vi "FeedBack.vi"() -> ()   [LabVIEW 2015]
doc: "This example performs a serial port write and a serial port read. The parameters set for the serial port must match the parameters of the connected instrument or device. The VISA Configure Serial Port VI sets the configuration parameters. The front panel displays the controls used to configure the basic parameters, such as baud rate, data bits, and parity. The VI passes the VISA resource name to other VIs that perform operations on that VISA resource. The VISA Write function sends a command to the serial device and the VISA Read function returns data based on the command. The VISA Close function then closes the reference to the serial device. It is important to close the reference; otherwise, further communication through that port might not be possible."
uses:
  support/Serial - Settings.ctl
  <vilib>/Instr/_visa.llb/VISA Configure Serial Port (Instr).vi
panel:
  out "AzimuthCurrentAngle":u16(knob) caption="ElevationCurrentAngle" scale=0.0..360.0
  in  "Parameter 2":u16
  in  "Azmuth WRITE PORT":refnum<visa-resource-name>="COM1"
  out "AzimuthDirection":string
  out "bytes written 2":u32
  out "Azmuth Encoder":string
  out "bytes read 2":u32
  out "hex integer string 4":string
  out "hex integer string 3":string
  in  "AzimuthRequiredAngle":u16=50
  in  "Azmuth READ PORT":refnum<visa-resource-name>="COM1"
  in  "Elevation WRITE PORT":refnum<visa-resource-name>="COM1"
  out "ElevationDirection":string
  out "bytes written":u32
  out "ElevationCurrentAngle":u16(knob) scale=0.0..360.0
  in  "ElevationRequiredAngle":u16=50
  out "hex integer string 2":string
  out "hex integer string":string
  in  "Parameter":u16
  in  "Combo Box":string(combo)="Get_Position"
  in  "Serial Settings":T1={"baud rate"=9600, "data bits"=8, "parity"=enum."None", "stop bits"=10, "flow control"=0} {"flow control" items=["None"=0, "XON/XOFF"=1, "RTS/CTS"=2, "DTR/DSR"=4]; "stop bits" items=["1.0"=10, "1.5"=15, "2.0"=20]; "data bits" min=5 max=8 step=1; "baud rate" items=["75"=75, "110"=110, "134"=134, "150"=150, "300"=300, "600"=600, "1200"=1200, "1800"=1800, "2400"=2400, "4800"=4800, "7200"=7200, "9600"=9600, "14400"=14400, "19200"=19200, "28800"=28800, "38400"=38400, "56000"=56000, "57600"=57600, "115200"=115200, "128000"=128000, "230400"=230400]}
  out "bytes read":u32
  in  "delay before read (ms)":u32=500
  out "Elevation Encoder":string
  in  "Elevation READ PORT":refnum<visa-resource-name>="COM1"
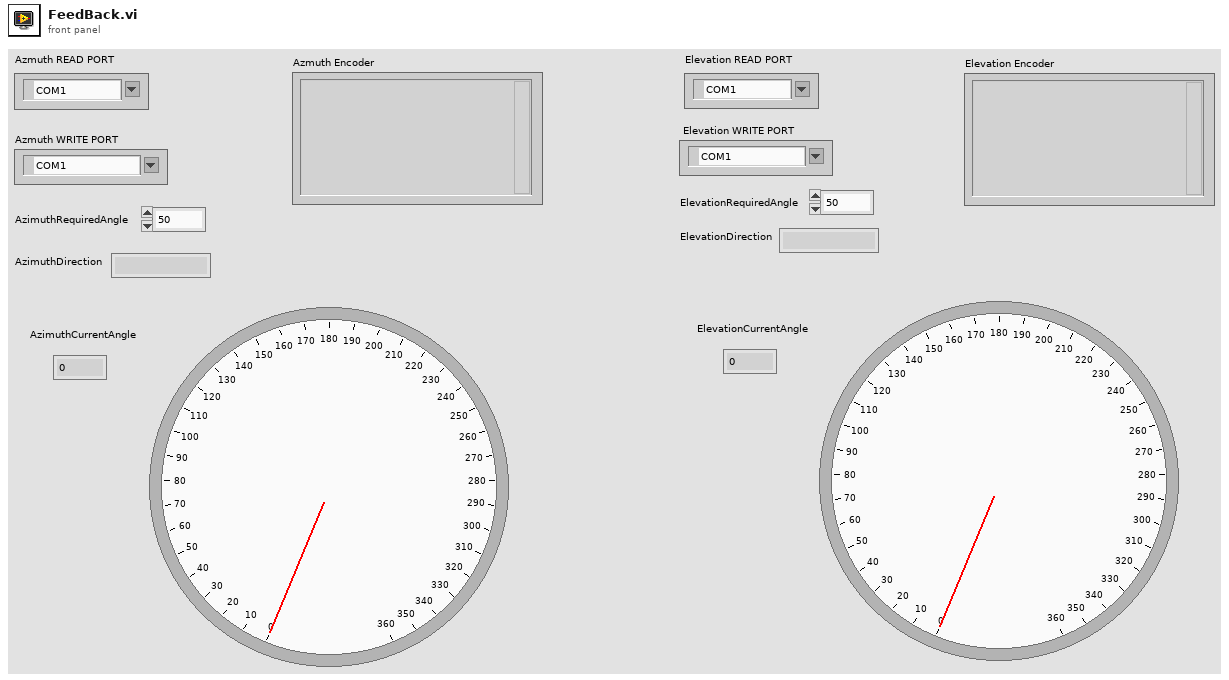
[diagram p1: front panel]
types:
  T1 = typedef "Serial - Settings.ctl" = cluster{"baud rate":u32, "data bits":u16, "parity":enum16{"None", "Odd", "Even", "Mark", "Space"}, "stop bits":u16, "flow control":u16}
  T2 = enum16{"big-endian, network order", "native, host order", "little-endian"}
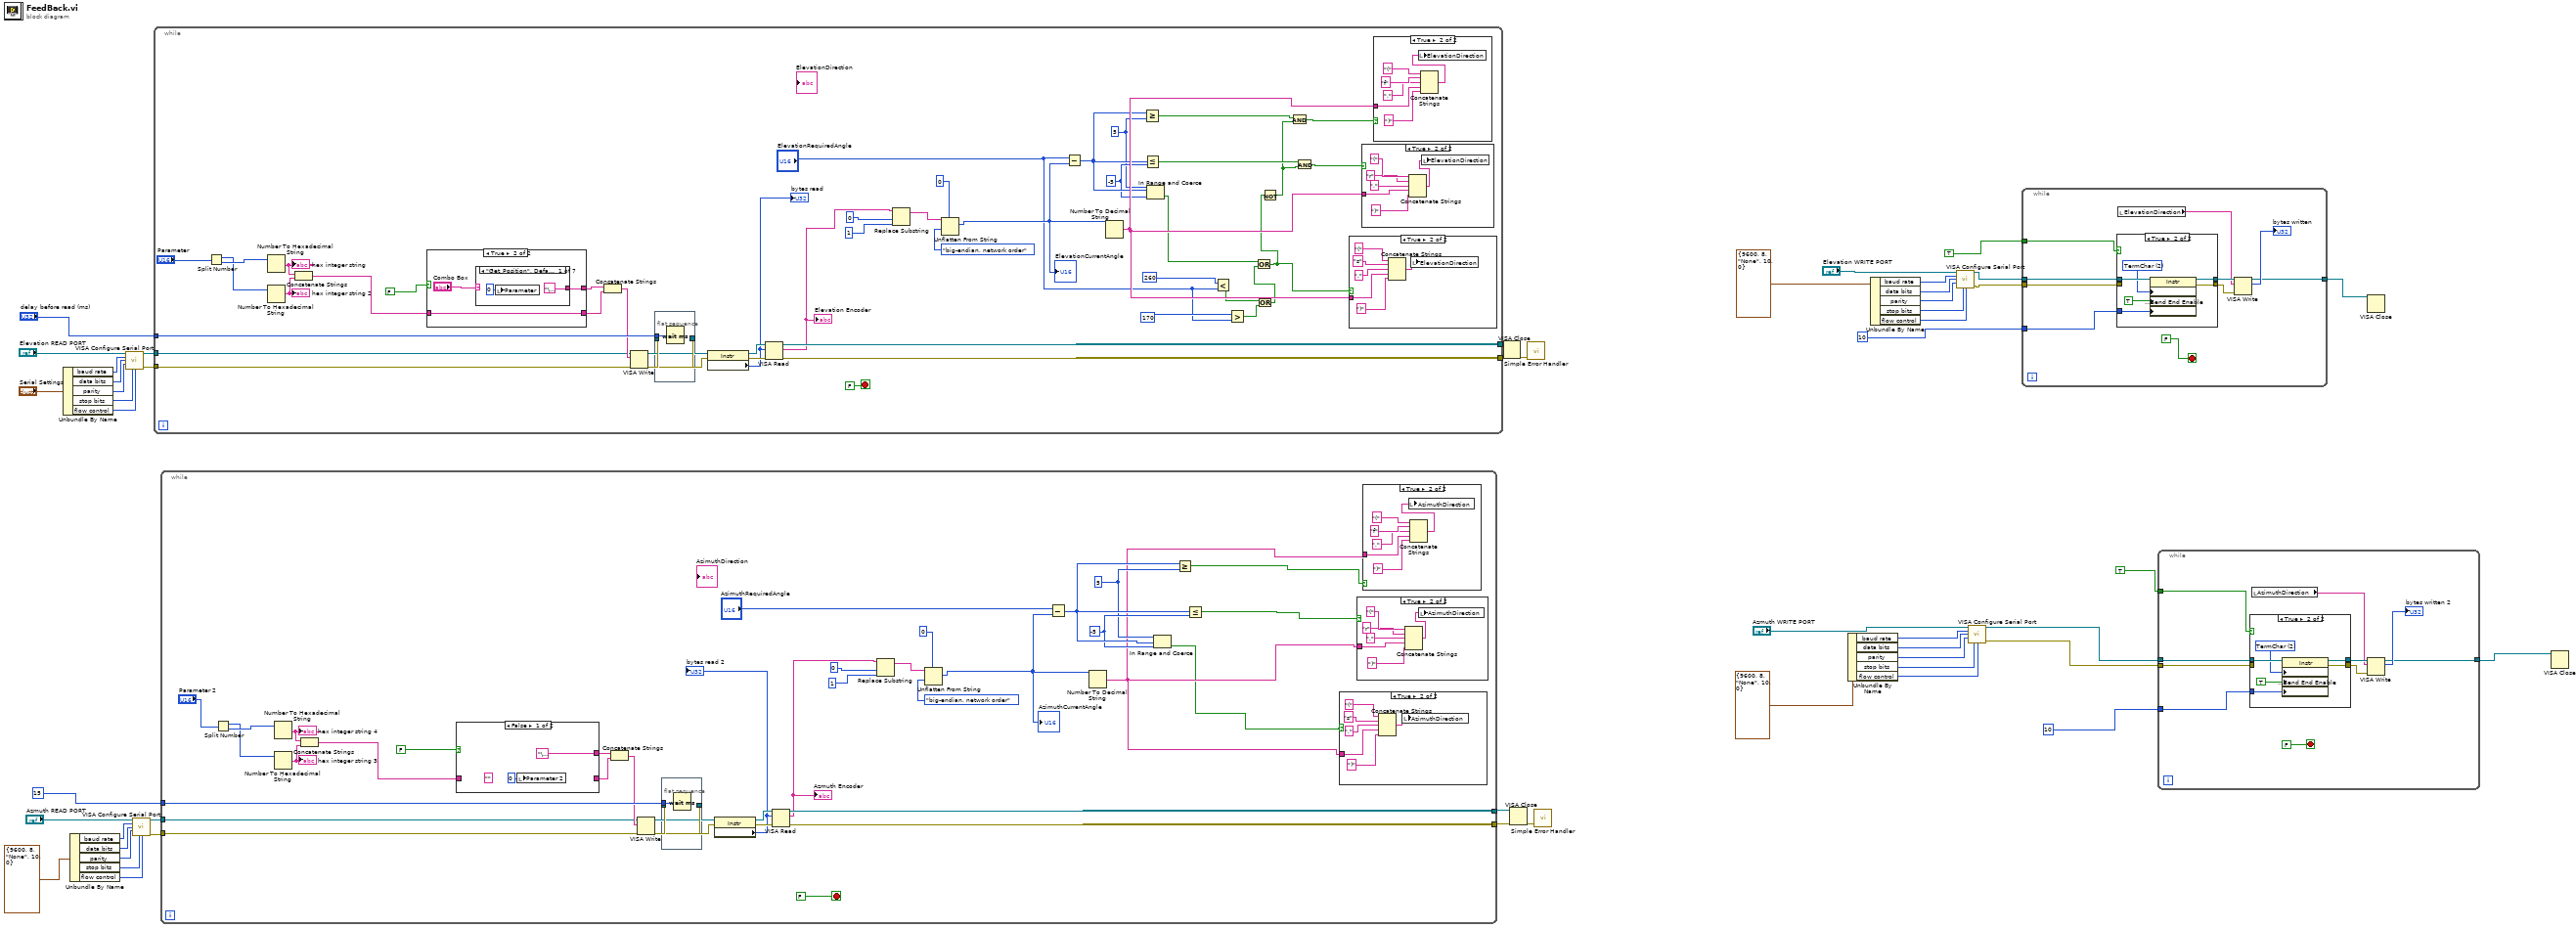
[diagram p0: block diagram]
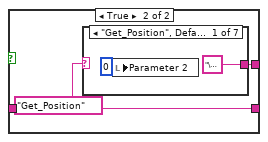
[diagram p6: hidden frame]
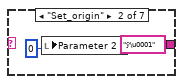
[diagram p7: hidden frame]
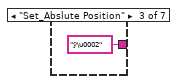
[diagram p8: hidden frame]
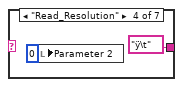
[diagram p9: hidden frame]
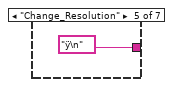
[diagram p10: hidden frame]
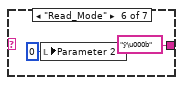
[diagram p11: hidden frame]
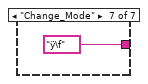
[diagram p12: hidden frame]
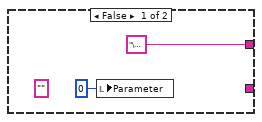
[diagram p17: hidden frame]
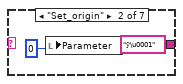
[diagram p18: hidden frame]
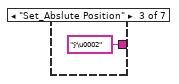
[diagram p19: hidden frame]
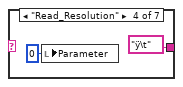
[diagram p20: hidden frame]
diagram:
  n1 = Unbundle By Name("Serial Settings") -> ("baud rate"=w45:u32, "data bits"=w44:u16, "parity"=w43:enum16{"None", "Odd", "Even", "Mark", "Space"}, "stop bits"=w42:u16, "flow control"=w41:u16)
  n2 = Unbundle By Name(T1 {"baud rate"=9600, "data bits"=8, "parity"=enum."None", "stop bits"=10, "flow control"=0} ("Serial Settings 2")) -> ("baud rate"=w20:u32, "data bits"=w19:u16, "parity"=w18:enum16{"None", "Odd", "Even", "Mark", "Space"}, "stop bits"=w17:u16, "flow control"=w16:u16)
  n3 = call-poly "VISA Configure Serial Port"("VISA resource name"="Elevation READ PORT", "baud rate (9600)"=w45, "data bits (8)"=w44, "parity (0:none)"=w43, "stop bits (10: 1 bit)"=w42, "flow control (0:none)"=w41) -> ("VISA resource name out"=w40:refnum<visa-resource-name>, "error out"=w39:errorcluster)  [unwired: 3 in, 5 out]
  n4 = call-poly "VISA Configure Serial Port"("VISA resource name"="Azmuth READ PORT", "baud rate (9600)"=w20, "data bits (8)"=w19, "parity (0:none)"=w18, "stop bits (10: 1 bit)"=w17, "flow control (0:none)"=w16) -> ("VISA resource name out"=w15:refnum<visa-resource-name>, "error out"=w14:errorcluster)  [unwired: 3 in, 5 out]
  n5 = while {
    tunnel: "delay before read (ms)" -> [w91]
    tunnel: w39 -> [w81]
    tunnel: [w97] -> w49
    tunnel: w40 -> [w82]
    tunnel: [w96] -> w48
    stop <- FALSE ("stop") stop-if-true
    w56 = -5
    w55 = 5
    n6 = Split Number(x="Parameter") -> (hi(x)=w77:u8, lo(x)=w78:u8)
    n7 = Number To Hexadecimal String(2:w78) -> (0:w76:string)  [unwired: 1 in]
    "hex integer string" <- w76
    n8 = Number To Hexadecimal String(2:w77) -> (0:w75:string)  [unwired: 1 in]
    "hex integer string 2" <- w75
    n9 = Concatenate Strings(w76, w75) -> (w79:string)
    n10 = case shown="True" FALSE ("Send command") {
      tunnel: ["\u001f" w120] -> w84
      tunnel: [_ w118] -> w83
      tunnel: w79 -> [_ w118]
      frame False {
        (unwired) "" ("Parameter")
        n11 = local write "Parameter"(u16 0 ("Parameter")) -> ()
      }
      frame True {
        n12 = case shown="\"Get_Position\", Default" "Combo Box" {
          tunnel: ["\u001f" "ÿ\u0001" "ÿ\u0002" "ÿ\t" "ÿ\n" "ÿ\u000b" "ÿ\f"] -> w120
          frame "Get_Position", Default {
            n13 = local write "Parameter"(u16 0 ("Parameter")) -> ()
          }
          frame "Set_origin" {
            n14 = local write "Parameter"(u16 0 ("Parameter")) -> ()
          }
          frame "Set_Abslute Position" {
          }
          frame "Read_Resolution" {
            n15 = local write "Parameter"(u16 0 ("Parameter")) -> ()
          }
          frame "Change_Resolution" {
          }
          frame "Read_Mode" {
            n16 = local write "Parameter"(u16 0 ("Parameter")) -> ()
          }
          frame "Change_Mode" {
          }
        }
      }
    }
    n17 = Concatenate Strings(w84, w83) -> (w85:string)
    n18 = VISA Write(VISA resource name=w82, write buffer=w85, error in (no error)=w81) -> (VISA resource name out=w93:refnum<visa-resource-name>, error out=w95:errorcluster)  [unwired: 1 out]
    n19 = flat-sequence {
      tunnel: w95 -> [w133]
      tunnel: [w133] -> w94
      tunnel: w93 -> [w132]
      tunnel: [w132] -> w92
      tunnel: w91 -> [w134]
      frame #0 {
        n20 = Wait (ms)(milliseconds to wait=w134) -> ()  [unwired: 1 out]
      }
    }
    n21 = property class="Instr"(reference=w92, error in=w94) -> (reference out=w90:refnum<visa-resource-name>, error out=w89:errorcluster, "Serial Settings:Number of Bytes at Serial Port"=w88:u32)
    "bytes read" <- w88
    n22 = VISA Read(VISA resource name=w90, byte count=w88, error in (no error)=w89) -> (VISA resource name out=w96:refnum<visa-resource-name>, read buffer=w69:string, error out=w97:errorcluster)  [unwired: 1 out]
    "Elevation Encoder" <- w69
    n23 = Replace Substring(2:1, 3:0, 5:w69) -> (1:w70:string)  [unwired: 1 in, 1 out]
    n24 = Unflatten From String(type=u16 0 ("I32"), binary string=w70, byte order (0:big-endian, network order)=T2."big-endian, network order" ("Byte Order 4")) -> (value=w58:u16)  [unwired: 2 in, 2 out]
    "ElevationCurrentAngle" <- w58
    n25 = Subtract(x="ElevationRequiredAngle", y=w58) -> (x-y=w57:i32)
    n26 = Number To Decimal String(number=w58) -> (decimal integer string=w68:string)  [unwired: 1 in]
    n27 = Greater Or Equal?(x=w57, y=w55) -> (x >= y?=w62:bool)
    n28 = Less Or Equal?(x=w57, y=w56) -> (x <= y?=w60:bool)
    n29 = In Range and Coerce(upper limit=w55, x=w57, lower limit=w56) -> (In Range?=w53:bool)  [unwired: 1 out]
    n30 = Less?(x=260, y="ElevationRequiredAngle") -> (x < y?=w65:bool)
    n31 = Greater?(x=170, y="ElevationRequiredAngle") -> (0:w64:bool)
    n32 = Or(x=w65, y=w64) -> (x .or. y?=w63:bool)
    n33 = Or(x=w53, y=w63) -> (x .or. y?=w52:bool)
    n34 = Not(x=w52) -> (.not. x?=w51:bool)
    n35 = And(x=w62, y=w51) -> (x .and. y?=w61:bool)
    n36 = And(x=w60, y=w51) -> (x .and. y?=w59:bool)
    n37 = case shown="True" w52 {
      tunnel: w68 -> [_ w99]
      frame False {
      }
      frame True {
        n38 = Concatenate Strings("(", "s", ",", w99, ")") -> (w100:string)
        n39 = local write "ElevationDirection"(w100) -> ()
      }
    }
    n40 = case shown="True" w59 {
      tunnel: w68 -> [_ w106]
      frame False {
      }
      frame True {
        n41 = Concatenate Strings("(", "r", ",", w106, ")") -> (w104:string)
        n42 = local write "ElevationDirection"(w104) -> ()
      }
    }
    n43 = case shown="True" w61 {
      tunnel: w68 -> [_ w112]
      frame False {
      }
      frame True {
        n44 = Concatenate Strings("(", "f", ",", w112, ")") -> (w110:string)
        n45 = local write "ElevationDirection"(w110) -> ()
      }
    }
  }
  n46 = while {
    tunnel: u32 15 ("delay before read (ms) 2") -> [w166]
    tunnel: w14 -> [w156]
    tunnel: [w172] -> w24
    tunnel: w15 -> [w157]
    tunnel: [w171] -> w23
    stop <- FALSE ("stop 3") stop-if-true
    w142 = -5
    w141 = 5
    n47 = Split Number(x="Parameter 2") -> (hi(x)=w153:u8, lo(x)=w154:u8)
    n48 = Number To Hexadecimal String(2:w154) -> (0:w152:string)  [unwired: 1 in]
    "hex integer string 4" <- w152
    n49 = Number To Hexadecimal String(2:w153) -> (0:w151:string)  [unwired: 1 in]
    "hex integer string 3" <- w151
    n50 = Concatenate Strings(w152, w151) -> (w155:string)
    n51 = case shown="False" FALSE ("Send command 2") {
      tunnel: ["\u001f" w195] -> w159
      tunnel: [_ w193] -> w158
      tunnel: w155 -> [_ w193]
      frame False {
        (unwired) "" ("Parameter")
        n52 = local write "Parameter 2"(u16 0 ("Parameter")) -> ()
      }
      frame True {
        n53 = case shown="\"Get_Position\", Default" "Get_Position" ("Combo Box 2") {
          tunnel: ["\u001f" "ÿ\u0001" "ÿ\u0002" "ÿ\t" "ÿ\n" "ÿ\u000b" "ÿ\f"] -> w195
          frame "Get_Position", Default {
            n54 = local write "Parameter 2"(u16 0 ("Parameter")) -> ()
          }
          frame "Set_origin" {
            n55 = local write "Parameter 2"(u16 0 ("Parameter")) -> ()
          }
          frame "Set_Abslute Position" {
          }
          frame "Read_Resolution" {
            n56 = local write "Parameter 2"(u16 0 ("Parameter")) -> ()
          }
          frame "Change_Resolution" {
          }
          frame "Read_Mode" {
            n57 = local write "Parameter 2"(u16 0 ("Parameter")) -> ()
          }
          frame "Change_Mode" {
          }
        }
      }
    }
    n58 = Concatenate Strings(w159, w158) -> (w160:string)
    n59 = VISA Write(VISA resource name=w157, write buffer=w160, error in (no error)=w156) -> (VISA resource name out=w168:refnum<visa-resource-name>, error out=w170:errorcluster)  [unwired: 1 out]
    n60 = flat-sequence {
      tunnel: w170 -> [w208]
      tunnel: [w208] -> w169
      tunnel: w168 -> [w207]
      tunnel: [w207] -> w167
      tunnel: w166 -> [w209]
      frame #0 {
        n61 = Wait (ms)(milliseconds to wait=w209) -> ()  [unwired: 1 out]
      }
    }
    n62 = property class="Instr"(reference=w167, error in=w169) -> (reference out=w165:refnum<visa-resource-name>, error out=w164:errorcluster, "Serial Settings:Number of Bytes at Serial Port"=w163:u32)
    "bytes read 2" <- w163
    n63 = VISA Read(VISA resource name=w165, byte count=w163, error in (no error)=w164) -> (VISA resource name out=w171:refnum<visa-resource-name>, read buffer=w140:string, error out=w172:errorcluster)  [unwired: 1 out]
    "Azmuth Encoder" <- w140
    n64 = Replace Substring(2:1, 3:0, 5:w140) -> (1:w145:string)  [unwired: 1 in, 1 out]
    n65 = Unflatten From String(type=u16 0 ("I32"), binary string=w145, byte order (0:big-endian, network order)=T2."big-endian, network order" ("Byte Order 4")) -> (value=w144:u16)  [unwired: 2 in, 2 out]
    "AzimuthCurrentAngle" <- w144
    n66 = Subtract(x="AzimuthRequiredAngle", y=w144) -> (x-y=w143:i32)
    n67 = Number To Decimal String(number=w144) -> (decimal integer string=w138:string)  [unwired: 1 in]
    n68 = In Range and Coerce(upper limit=w141, x=w143, lower limit=w142) -> (In Range?=w137:bool)  [unwired: 1 out]
    n69 = Greater Or Equal?(x=w143, y=w141) -> (x >= y?=w136:bool)
    n70 = Less Or Equal?(x=w143, y=w142) -> (x <= y?=w135:bool)
    n71 = case shown="True" w137 {
      tunnel: w138 -> [_ w174]
      frame False {
      }
      frame True {
        n72 = Concatenate Strings("(", "s", ",", w174, ")") -> (w175:string)
        n73 = local write "AzimuthDirection"(w175) -> ()
      }
    }
    n74 = case shown="True" w135 {
      tunnel: w138 -> [_ w181]
      frame False {
      }
      frame True {
        n75 = Concatenate Strings("(", "r", ",", w181, ")") -> (w179:string)
        n76 = local write "AzimuthDirection"(w179) -> ()
      }
    }
    n77 = case shown="True" w136 {
      tunnel: w138 -> [_ w187]
      frame False {
      }
      frame True {
        n78 = Concatenate Strings("(", "f", ",", w187, ")") -> (w185:string)
        n79 = local write "AzimuthDirection"(w185) -> ()
      }
    }
  }
  n80 = VISA Close(VISA resource name=w48, error in (no error)=w49) -> (error out=w47:errorcluster)
  n81 = VISA Close(VISA resource name=w23, error in (no error)=w24) -> (error out=w22:errorcluster)
  n82 = call <vilib>:"Simple Error Handler.vi"("error in (no error)"=w47) -> ()  [unwired: 1 in, 8 out]
  n83 = call <vilib>:"Simple Error Handler.vi"("error in (no error)"=w22) -> ()  [unwired: 1 in, 8 out]
  n84 = Unbundle By Name(T1 {"baud rate"=9600, "data bits"=8, "parity"=enum."None", "stop bits"=10, "flow control"=0} ("Serial Settings (write) 2")) -> ("baud rate"=w10:u32, "data bits"=w9:u16, "parity"=w8:enum16{"None", "Odd", "Even", "Mark", "Space"}, "stop bits"=w7:u16, "flow control"=w6:u16)
  n85 = Unbundle By Name(T1 {"baud rate"=9600, "data bits"=8, "parity"=enum."None", "stop bits"=10, "flow control"=0} ("Serial Settings (write)")) -> ("baud rate"=w35:u32, "data bits"=w34:u16, "parity"=w33:enum16{"None", "Odd", "Even", "Mark", "Space"}, "stop bits"=w32:u16, "flow control"=w31:u16)
  n86 = call-poly "VISA Configure Serial Port"("VISA resource name"="Elevation WRITE PORT", "baud rate (9600)"=w35, "data bits (8)"=w34, "parity (0:none)"=w33, "stop bits (10: 1 bit)"=w32, "flow control (0:none)"=w31) -> ("VISA resource name out"=w29:refnum<visa-resource-name>, "error out"=w28:errorcluster)  [unwired: 3 in, 5 out]
  n87 = call-poly "VISA Configure Serial Port"("VISA resource name"="Azmuth WRITE PORT", "baud rate (9600)"=w10, "data bits (8)"=w9, "parity (0:none)"=w8, "stop bits (10: 1 bit)"=w7, "flow control (0:none)"=w6) -> ("VISA resource name out"=w5:refnum<visa-resource-name>, "error out"=w4:errorcluster)  [unwired: 3 in, 5 out]
  n88 = while {
    tunnel: TRUE ("End Write on Termination Character?") -> [w214]
    tunnel: w29 -> [w213]
    tunnel: w28 -> [w212]
    tunnel: u8 10 ("Termination Character") -> [w211]
    tunnel: [w210] -> w26
    stop <- FALSE ("stop 2") stop-if-true
    n89 = case shown="True" w214 {
      tunnel: w213 -> [w220 w227]
      tunnel: w212 -> [w221 _]
      tunnel: [w220 w226] -> w218
      tunnel: [w221 w225] -> w217
      tunnel: w211 -> [_ w223]
      frame False {
      }
      frame True {
        w224 = u16 2 items=["None", "LastBit", "TermChar", "Break"] ("Serial Settings:Serial End Mode for Writes")
        n90 = property class="Instr"(reference=w227, "Serial Settings:End Mode for Writes"=w224, "Message Based Settings:Send End Enable"=TRUE, "Message Based Settings:Termination Character"=w223) -> (reference out=w226:refnum<visa-resource-name>, error out=w225:errorcluster)  [unwired: 1 in]
      }
    }
    n91 = local read "ElevationDirection"() -> (w215:string)
    n92 = VISA Write(VISA resource name=w218, write buffer=w215, error in (no error)=w217) -> (VISA resource name out=w210:refnum<visa-resource-name>, return count=→"bytes written":u32)  [unwired: 1 out]
  }
  n93 = while {
    tunnel: TRUE ("End Write on Termination Character? 2") -> [w233]
    tunnel: w5 -> [w232]
    tunnel: w4 -> [w231]
    tunnel: u8 10 ("Termination Character 2") -> [w230]
    tunnel: [w229] -> w2
    stop <- FALSE ("stop 3") stop-if-true
    n94 = case shown="True" w233 {
      tunnel: w232 -> [w238 w245]
      tunnel: w231 -> [w239 _]
      tunnel: [w238 w244] -> w236
      tunnel: [w239 w243] -> w235
      tunnel: w230 -> [_ w241]
      frame False {
      }
      frame True {
        w242 = u16 2 items=["None", "LastBit", "TermChar", "Break"] ("Serial Settings:Serial End Mode for Writes")
        n95 = property class="Instr"(reference=w245, "Serial Settings:End Mode for Writes"=w242, "Message Based Settings:Send End Enable"=TRUE, "Message Based Settings:Termination Character"=w241) -> (reference out=w244:refnum<visa-resource-name>, error out=w243:errorcluster)  [unwired: 1 in]
      }
    }
    n96 = local read "AzimuthDirection"() -> (w234:string)
    n97 = VISA Write(VISA resource name=w236, write buffer=w234, error in (no error)=w235) -> (VISA resource name out=w229:refnum<visa-resource-name>, return count=→"bytes written 2":u32)  [unwired: 1 out]
  }
  n98 = VISA Close(VISA resource name=w26) -> ()  [unwired: 1 in, 1 out]
  n99 = VISA Close(VISA resource name=w2) -> ()  [unwired: 1 in, 1 out]
